vi "Load GT-BIRD.vi"(8 "error in (no error)":errorcluster, 11 "Name":string="BIRD-3D") -> (0 "error out":errorcluster, 3 "BIRD-3D output":T1)   [LabVIEW 2013]
uses:
  BIRD-3D.ctl
  <vilib>/picture/3D Picture Control/Object/Create Object (name).vi
  <vilib>/picture/3D Picture Control/NI_3D Picture Control.lvlib
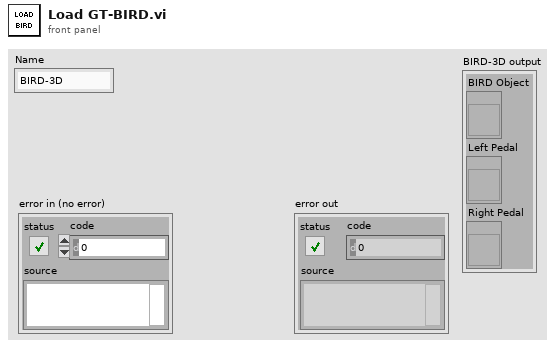
[diagram p1: front panel]
types:
  T1 = typedef "BIRD-3D.ctl" = cluster{"BIRD Object":refnum<vi>, "Left Pedal":refnum<vi>, "Right Pedal":refnum<vi>}
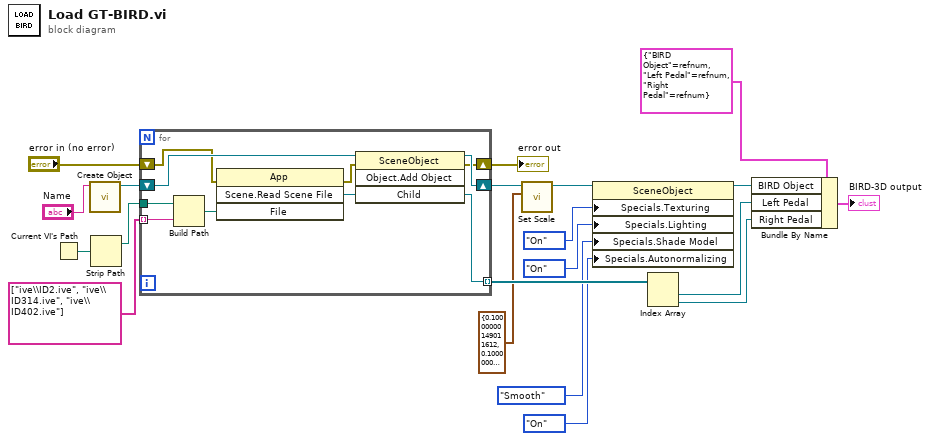
[diagram p0: block diagram]
diagram:
  n1 = Current VI's Path() -> (path=w20:path)
  n2 = call-poly <vilib>:"Create Object.vi"("Name"="Name") -> ("Scene:New Object"=w17:refnum<vi>)  [unwired: 9 in, 1 out]
  n3 = Strip Path(path=w20) -> (stripped path=w19:path)  [unwired: 1 out]
  n4 = for {
    tunnel: w19 -> [w30]
    tunnel: string[] ["ive\\ID2.ive", "ive\\ID314.ive", "ive\\ID402.ive"] -> [w29] mode=indexing
    shift-right: [w26] -> w8
    shift-left: w17 -> [w27]
    tunnel: [w24] -> w15 mode=indexing
    shift-right: [w21] -> w9
    shift-left: "error in (no error)" -> [w23]
    n5 = Build Path(base path=w30, name or relative path=w29) -> (appended path=w28:path)
    n6 = invoke class="App" method="Scene.Read Scene File"(error in=w23, "File"=w28) -> (error out=w22:errorcluster, "Scene.Read Scene File"=w25:refnum<vi>)  [unwired: 2 in, 2 out]
    n7 = invoke class="SceneObject" method="Object.Add Object"(reference=w27, error in=w22, "Child"=w25) -> (reference out=w26:refnum<vi>, error out=w21:errorcluster, "Child"=w24:refnum<vi>)  [unwired: 1 in, 1 out]
  }
  "error out" <- w9
  n8 = call <vilib>:"Set Scale.vi"("Scale"=cluster{"X":sgl, "Y":sgl, "Z":sgl} {"X"=0.1, "Y"=0.1, "Z"=0.1}, "Scene Object"=w8) -> ("Scaled Object"=w2:refnum<vi>)  [unwired: 8 in, 1 out]
  n9 = property class="SceneObject"(reference=w2, "Specials.Texturing"=enum16{"Inherit Value", "Off", "On"}."On" ("Specials:Texturing"), "Specials.Lighting"=enum16{"Inherit Value", "Off", "On"}."On" ("Specials:Lighting"), "Specials.Shade Model"=enum16{"Inherit Value", "Flat", "Smooth"}."Smooth" ("Specials:Shade Model"), "Specials.Autonormalizing"=enum16{"Inherit Value", "Off", "On"}."On" ("Specials:Autonormalizing")) -> (reference out=w1:refnum<vi>)  [unwired: 1 in, 1 out]
  n10 = Index Array(array=w15) -> (element #1=w14:refnum<vi>, element #2=w13:refnum<vi>)  [unwired: 2 in]
  n11 = Bundle By Name(cluster=T1 {"BIRD Object"=refnum, "Left Pedal"=refnum, "Right Pedal"=refnum} ("BIRD-3D"), "BIRD Object"=w1, "Left Pedal"=w14, "Right Pedal"=w13) -> (→"BIRD-3D output":T1)
